vi "MQTT_Subscribe.vi"(8 "error in (no error)":errorcluster, 9 "Message ID":u16=10 format="%x", 10 "Subscription Info Array":cluster{"Topic":string, "QoS":T2}[](array[cluster])=[{"Topic"="a/b", "QoS"=enum."At least once"}], 11 "SSL_Connection":T1) -> (0 "error out":errorcluster, 3 "SSL_Connection":T1)   [LabVIEW 2018, in "AWS_IoT.lvlib"]
doc: "This VI subscribes the client to a selected topic. The client now can read published messages for the topic. \n\n© 2015 - daq.io, LLC - Peter Adelhardt"
uses:
  AWS_IoT.lvlib
  Controls/QoS.ctl
  Controls/SSL_Connection.ctl
  Controls/MessageType.ctl
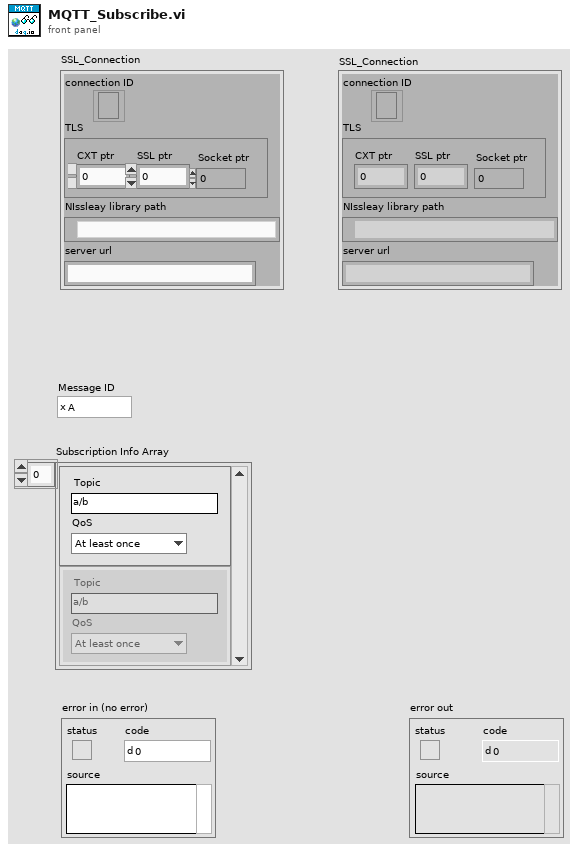
[diagram p1: front panel]
types:
  T1 = typedef "AWS_IoT.lvlib/SSL_Connection.ctl" = cluster{"connection ID":refnum<k5>, "TLS":cluster{"CXT ptr":i32, "SSL ptr":i32, "Socket ptr":i32}, "NIssleay library path":path, "server url":string}
  T2 = typedef "AWS_IoT.lvlib/QoS.ctl" = enum8{"At most once", "At least once", "Exactly once", "Reserved"}
  T3 = typedef "AWS_IoT.lvlib/MessageType.ctl" = enum32{"Reserved", "CONNECT", "CONNACK", "PUBLISH", "PUBACK", "PUBREC", "PUBREL", "PUBCOMP", "SUBSCRIBE", "SUBACK", "UNSUBSCRIBE", "UNSUBACK", "PINGREQ", "PINGRESP", "DISCONNECT", "Reserved2"}
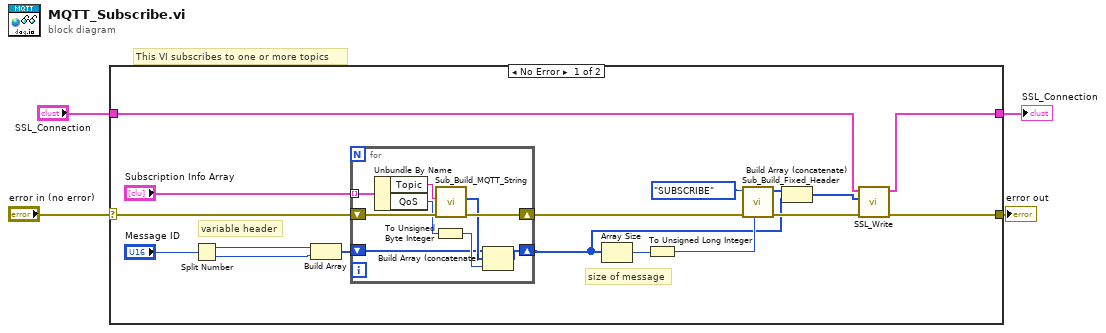
[diagram p0: block diagram]
diagram:
  # "This VI subscribes to one or more topics"
  n1 = case shown="No Error" "error in (no error)" {
    selector: "error in (no error)" -> [w15 w32]
    tunnel: [w9 w32] -> w3
    tunnel: "SSL_Connection" -> [w6 w31]
    tunnel: [w5 w31] -> w1
    frame No Error {
      # "variable header"
      # "size of message"
      n2 = Split Number(x="Message ID") -> (hi(x)=w18:u8, lo(x)=w17:u8)
      n3 = Build Array(w18, w17) -> (w13:u8[])
      n4 = for {
        tunnel: "Subscription Info Array" -> [w30] mode=indexing
        shift-right: [w27] -> w12
        shift-left: w15 -> [w28]
        shift-right: [w23] -> w8
        shift-left: w13 -> [w22]
        n5 = Unbundle By Name(w30) -> ("Topic"=w29:string, "QoS"=w26:T2)
        n6 = To Unsigned Byte Integer(number=w26) -> (unsigned 8bit integer=w24:u8)
        n7 = call "Sub_Build_MQTT_String.vi"("error in (no error)"=w28, "String to be encoded"=w29) -> ("error out"=w27:errorcluster, "UTF8 Byte Array"=w25:u8[])  [unwired: 8 in]
        n8 = Build Array (concatenate)(w22, w25, w24) -> (w23:u8[])
      }
      n9 = Array Size(array=w8) -> (size(s)=w20:i32)
      n10 = To Unsigned Long Integer(number=w20) -> (unsigned 32bit integer=w21:u32)
      n11 = call "Sub_Build_Fixed_Header.vi"("Remaining Length"=w21, "error in (no error)"=w12, "MessageType"=MessageType."SUBSCRIBE") -> ("error out"=w10:errorcluster, "Fixed Header"=w19:u8[])  [unwired: 7 in]
      n12 = Build Array (concatenate)(w19, w8) -> (w11:u8[])
      n13 = call "SSL_Write.vi"("error in (no error)"=w10, "data in"=w11, "SSL_Connection"=w6) -> ("error out"=w9:errorcluster, "SSL_Connection"=w5:T1)  [unwired: 7 in]
    }
    frame Error {
    }
  }
  "error out" <- w3
  "SSL_Connection" <- w1
